vi "Filter_default value.vi"() -> (1 "Filter Default Value":string)   [LabVIEW 2023]
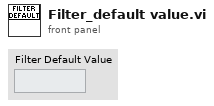
[diagram p1: front panel]
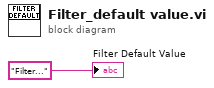
[diagram p0: block diagram]
diagram:
  "Filter Default Value" <- "Filter..." ("Filter Default Value")
